vi "Array To Autonomous Commands.vi"(2 "Which":dbl, 3 "Input Array":string[][][](array[string])) -> (0 "Float Output Array":dbl[](array[numeric]), 1 "String Output Array":string[](array[string]))   [LabVIEW 2015]
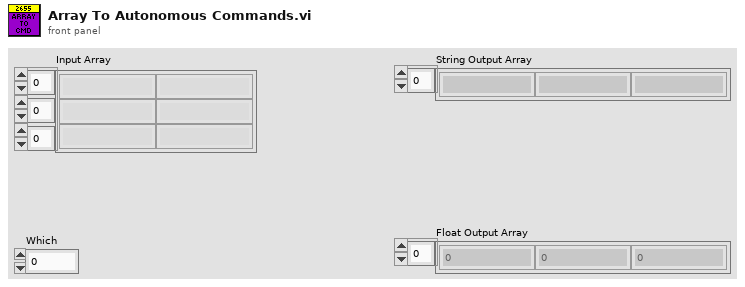
[diagram p1: front panel]
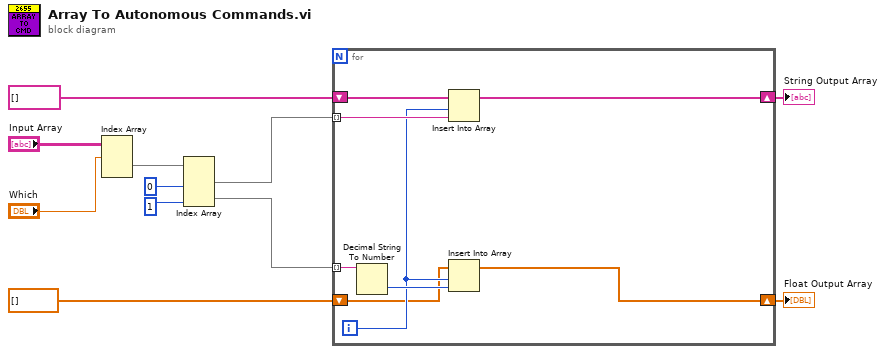
[diagram p0: block diagram]
diagram:
  n1 = Index Array(array="Input Array", index (dim 0)="Which") -> (element=w9:string[][])  [unwired: 2 in]
  n2 = Index Array(array=w9, index (col) #1=0, index (col) #2=1) -> (element #1=w6:string[], element #2=w5:string[])  [unwired: 2 in]
  n3 = for {
    tunnel: w6 -> [w19] mode=indexing
    tunnel: w5 -> [w16] mode=indexing
    shift-right: [w17] -> w1
    shift-left: string[] [] ("String Output Array 2") -> [w18]
    shift-right: [w12] -> w2
    shift-left: dbl[] [] ("Float Output Array") -> [w13]
    i -> [w14]
    n4 = Decimal String To Number(string=w16) -> (number=w15:i32)  [unwired: 2 in, 1 out]
    n5 = Insert Into Array(array=w18, index=w14, new element=w19) -> (w17:string[])
    n6 = Insert Into Array(array=w13, index=w14, new element=w15) -> (w12:dbl[])
  }
  "Float Output Array" <- w2
  "String Output Array" <- w1
